vi "setFileName.vi"(3 "extension":u16(ring) items=[".txt", ".tiff"], 4 "file_name":string, 5 "base_path":path) -> (2 "path_filename":path)   [LabVIEW 2018]
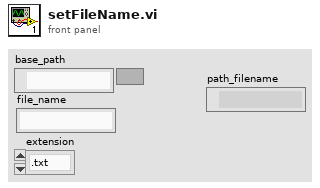
[diagram p1: front panel]
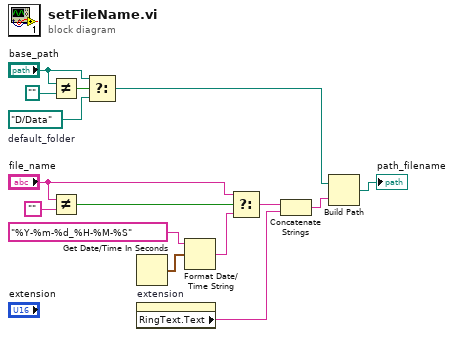
[diagram p0: block diagram]
diagram:
  w9 = path "D:/Data"  # default_folder
  n1 = Not Equal?(x="base_path", y=path "") -> (x != y?=w10:bool)
  n2 = Not Equal?(x="file_name", y="") -> (x != y?=w5:bool)
  n3 = Select(t="base_path", s=w10, f=w9) -> (s? t:f=w7:path)
  n4 = Get Date/Time In Seconds() -> (seconds since 1Jan1904=w12:timestamp)
  n5 = property on="extension" class="Ring (strict)"() -> ("RingText.Text"=w14:string)  [unwired: 2 in, 2 out]
  n6 = Format Date/Time String(time format string (%c)="%Y-%m-%d_%H-%M-%S", seconds (now)=w12) -> (date/time string=w4:string)  [unwired: 1 in]
  n7 = Select(t="file_name", s=w5, f=w4) -> (s? t:f=w3:string)
  n8 = Concatenate Strings(w3, w14) -> (w2:string)
  n9 = Build Path(base path=w7, name or relative path=w2) -> (appended path=→"path_filename":path)
